vi "ImageColorRgbaU64ToArray.vi"(8 "error in":errorcluster, 11 "Image Reference In":T3) -> (0 "error out":errorcluster, 2 "Pixel":T1[][](array[typedef]), 3 "Image Reference Out":T3)   [LabVIEW 2024, in "OpenLvVision_Image.lvlib" / "DataAccess.lvlib"]
doc: "Copies the pixel into an 2D array without an border."
uses:
  DataAccess.lvlib
  Management/TypeDef/Image.ctl
  TypeDef/RectangleI32.ctl
  Management/Management.lvlib
panel:
  in  "Optional Rectangle":T2
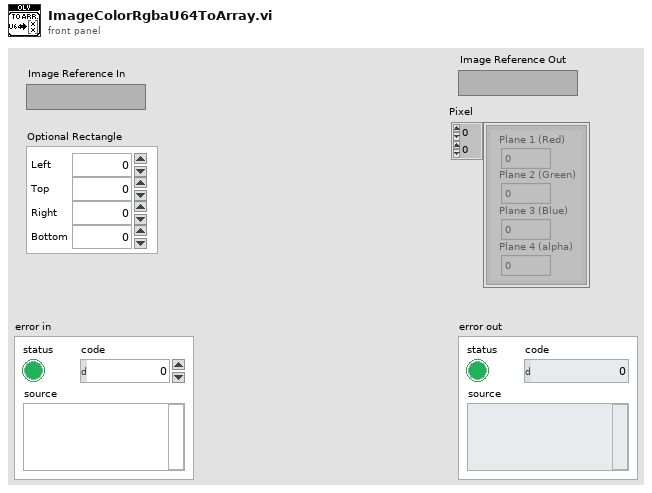
[diagram p1: front panel]
types:
  T1 = typedef "Color (U64)" = cluster{"Plane 3 (Blue)":u16, "Plane 2 (Green)":u16, "Plane 1 (Red)":u16, "Plane 4 (alpha)":u16}
  T2 = typedef "OpenLvVision_Image.lvlib/DataAccess.lvlib/RectangleI32.ctl" = cluster{"Left":i32, "Top":i32, "Right":i32, "Bottom":i32}
  T3 = typedef "OpenLvVision_Image.lvlib/Management.lvlib/Image.ctl" = refnum<image>
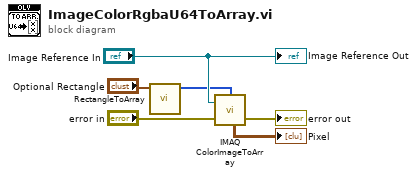
[diagram p0: block diagram]
diagram:
  n1 = call "RectangleToArray.vi"("Optional Rectangle"="Optional Rectangle") -> ("Array"=w2:i32[])  [unwired: 10 in]
  n2 = call "IMAQ ColorImageToArray"("Optional Rectangle"=w2, "Image"="Image Reference In", "error in (no error)"="error in") -> ("error out"=→"error out":errorcluster, "Image Pixels (U64)"=→"Pixel":T1[][])  [unwired: 1 in, 1 out]
  "Image Reference Out" <- "Image Reference In"
